vi "Configure Glitch Trigger Source [GT].vi"(0 "CS++Scope":refnum<class "CS++Scope.lvclass">, 1 "trigger source (\"CHANNEL1\")":string(combo)="CHANNEL1", 2 "trigger level (0.0 V)":dbl[unit] format="%.3f", 3 "glitch width (10 ms)":dbl[unit]=1e-05 format="%^.2e", 4 "glitch polarity (Positive)":i32(ring)=1 items=["Positive"=1, "Negative"=2, "Either"=3], 5 "error in (no error)":errorcluster, 6 "glitch condition (Less Than)":i32(ring)=1 items=["Less Than"=1, "Greater Than"=2]) -> (14 "CS++Scope out":refnum<class "CS++Scope.lvclass">, 19 "error out":errorcluster)   [LabVIEW 2015, in "CS++Scope.lvlib" / "CS++Scope.lvclass"]
doc: "This VI configures the glitch trigger. A glitch trigger occurs when the trigger signal has a pulse with a width that is less than or greater than the glitch width. You specifiy which comparison criterion to use with the glitchCondition parameter. You specifiy the glitch width in the glitchWidth parameter. You specifiy the polarity of the pulse with the glitchPolarity parameter. The trigger does not actually occur until the edge of a pulse that corresponds to the glitchWidth and glitchPolarity crosses the threshold the end-user specifies in the triggerLevel parameter.\n\nNote:\nThis VI affects instrument behavior only if the trigger type is IVISCOPE_VAL_GLITCH_TRIGGER. Call the IviScope Configure Trigger and IviScope Configure Trigger Coupling VIs to set the trigger type and trigger coupling before calling this VI."
uses:
  CS++Scope.lvclass
  CSPP_Core/Classes/CS++ProcessVariables/ProcessVariable/PV.lvclass
  PV-Enum.ctl
  CS++Scope.lvclass/CS++Scope.ctl
  CSPP_Core/Classes/CS++ProcessVariables/ProcessVariable/PV.lvclass/PV.ctl
  CSPP_Core/Classes/CS++ProcessVariables/ProcessVariable/Write Data.vi
  CSPP_Core/Classes/CS++ProcessVariables/ProcessVariable/Write Timestamp.vi
  CSPP_Core/Classes/CS++ProcessVariables/ProcessVariable/Write Quality.vi
  CSPP_Core/Classes/CS++ProcessVariables/ProcessVariable/Write status.vi
  CSPP_Core/Classes/CS++ProcessVariables/PVConnection/PVConnection.lvclass
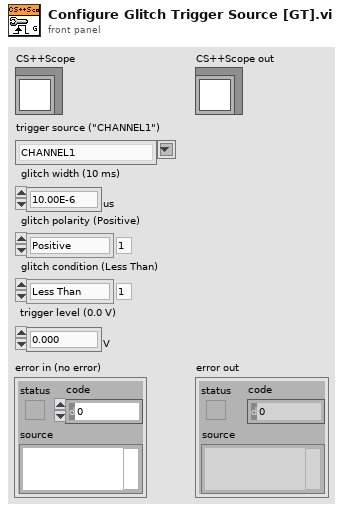
[diagram p1: front panel]
types:
  T1 = typedef "CS++Scope.lvlib/CS++Scope.lvclass/PV-Enum.ctl" = enum16{"ActualSampleRate", "TimePerRecord", "AcquisitionStartTime", "TriggerLevel", "GlitchWidth", "LowReference", "MidReference", "HighReference", "RuntLowThreshold", "RuntHighThreshold", "TriggerHoldoff", "WidthLowThreshold", "WidthHighThreshold", "AcquisitionStatus", "ActualRecordLength", "ActualSampleMode", "ACLineTriggerSlope", "MinRecordLength", "AcquisitionType", "TriggerSlope", "GlitchCondition", "GlitchPolarity", "InterpolationMethod", "NumberOfAverages", "NumberOfEnvelopes", "TriggerType", "TriggerCoupling", "TriggerModifier", "TVLineNumber", "TVEvent", "TVTriggerPolarity", "TVSignalFormat", "WidthCondition", "WidthPolarity", "MeasurementDone", "ContinousAcquisition", "TriggerSource", "Waveform", "ActualTimeIncrement"}
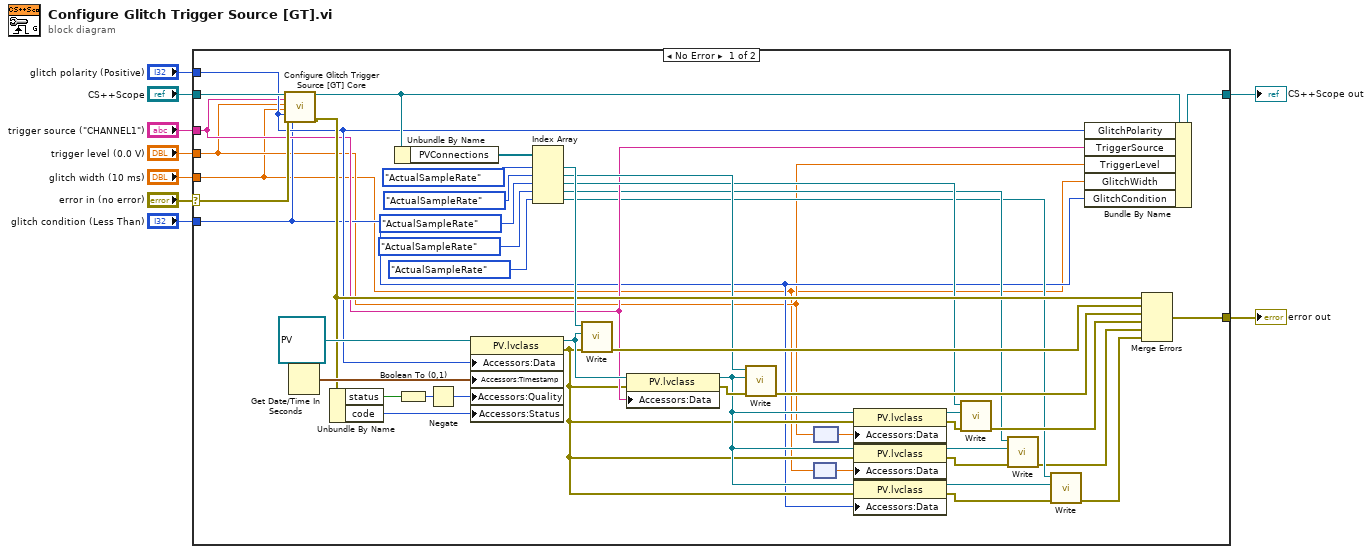
[diagram p0: block diagram]
diagram:
  n1 = case shown="No Error" "error in (no error)" {
    selector: "error in (no error)" -> [w30 w56]
    tunnel: [w29 w56] -> w8
    tunnel: [w31 w55] -> w2
    tunnel: "CS++Scope" -> [w32 w55]
    tunnel: "trigger source (\"CHANNEL1\")" -> [w25 _]
    tunnel: "trigger level (0.0 V)" -> [w13 _]
    tunnel: "glitch width (10 ms)" -> [w10 _]
    tunnel: "glitch polarity (Positive)" -> [w26 _]
    tunnel: "glitch condition (Less Than)" -> [w14 _]
    frame No Error {
      n2 = call-dynamic "Configure Glitch Trigger Source [GT] Core.vi"("CS++Scope"=w32, "trigger source (\"CHANNEL1\")"=w25, "trigger level (0.0 V)"=w13, "glitch width (10 ms)"=w10, "glitch polarity (Positive)"=w26, "error in (no error)"=w30, "glitch condition (Less Than)"=w14) -> ("CS++Scope out"=w44:refnum<class "CS++Scope.lvclass">, "error out"=w43:errorcluster)  [unwired: 11 in]
      n3 = Get Date/Time In Seconds() -> (seconds since 1Jan1904=w49:timestamp)
      n4 = Unbundle By Name(w43) -> ("status"=w52:bool, "code"=w53:i32)
      n5 = Unbundle By Name(w44) -> ("PVConnections"=w48:refnum<class "PVConnection.lvclass">[])
      n6 = Boolean To (0,1)(Boolean=w52) -> (0, 1=w51:i16)
      n7 = Negate(x=w51) -> (-x=w50:i16)
      n8 = property class="PV.lvclass"(reference=refnum<class "PV.lvclass"> refnum ("CS++ProcessVariables.lvlib:PV.lvclass"), "Accessors:Data"=w26, "Accessors:Timestamp"=w49, "Accessors:Quality"=w50, "Accessors:Status"=w53) -> (reference out=w38:refnum<class "PV.lvclass">, error out=w17:errorcluster)  [unwired: 1 in]
      n9 = Index Array(array=w48, index #1=PV-Enum."ActualSampleRate" ("PV-Enum"), index #2=PV-Enum."ActualSampleRate" ("PV-Enum"), index #3=PV-Enum."ActualSampleRate" ("PV-Enum"), index #4=PV-Enum."ActualSampleRate" ("PV-Enum"), index #5=PV-Enum."ActualSampleRate" ("PV-Enum")) -> (element #1=w46:refnum<class "PVConnection.lvclass">, element #2=w36:refnum<class "PVConnection.lvclass">, element #3=w34:refnum<class "PVConnection.lvclass">, element #4=w20:refnum<class "PVConnection.lvclass">, element #5=w19:refnum<class "PVConnection.lvclass">)
      n10 = call "Write.vi"("error in (no error)"=w17, "PV"=w38, "PVConnection in"=w46) -> ("error out"=w45:errorcluster)  [unwired: 7 in, 1 out]
      n11 = property class="PV.lvclass"(reference=w38, error in=w17, "Accessors:Data"=w25) -> (reference out=w18:refnum<class "PV.lvclass">, error out=w37:errorcluster)
      n12 = call "Write.vi"("error in (no error)"=w37, "PV"=w18, "PVConnection in"=w36) -> ("error out"=w40:errorcluster)  [unwired: 7 in, 1 out]
      n13 = node(w13) -> (w12:dbl)
      n14 = node(w10) -> (w11:dbl)
      n15 = property class="PV.lvclass"(reference=w18, error in=w17, "Accessors:Data"=w12) -> (reference out=w35:refnum<class "PV.lvclass">, error out=w33:errorcluster)
      n16 = property class="PV.lvclass"(reference=w18, error in=w17, "Accessors:Data"=w11) -> (reference out=w24:refnum<class "PV.lvclass">, error out=w23:errorcluster)
      n17 = property class="PV.lvclass"(reference=w18, error in=w17, "Accessors:Data"=w14) -> (reference out=w22:refnum<class "PV.lvclass">, error out=w21:errorcluster)
      n18 = call "Write.vi"("error in (no error)"=w33, "PV"=w35, "PVConnection in"=w34) -> ("error out"=w39:errorcluster)  [unwired: 7 in, 1 out]
      n19 = call "Write.vi"("error in (no error)"=w23, "PV"=w24, "PVConnection in"=w20) -> ("error out"=w16:errorcluster)  [unwired: 7 in, 1 out]
      n20 = call "Write.vi"("error in (no error)"=w21, "PV"=w22, "PVConnection in"=w19) -> ("error out"=w15:errorcluster)  [unwired: 7 in, 1 out]
      n21 = Bundle By Name(cluster=w44, "GlitchPolarity"=w26, "TriggerSource"=w25, "TriggerLevel"=w13, "GlitchWidth"=w10, "GlitchCondition"=w14) -> (w31:refnum<class "CS++Scope.lvclass">)
      n22 = Merge Errors(w43, w45, w40, w39, w16, w15) -> (w29:errorcluster)
    }
    frame Error {
    }
  }
  "error out" <- w8
  "CS++Scope out" <- w2
